vi "preliminaries.vi"(5 "Version":string, 6 "error in":errorcluster, 9 "control cluster":T1) -> (0 "error out":errorcluster, 1 "timing source out":string, 3 "reference cluster out":T2, 4 "error event refnum":refnum<event-registration>)   [LabVIEW 2016]
uses:
  Type Definitions/reference_cluster.ctl
  Type Definitions/vars_settings.ctl
  Type Definitions/stim_type.ctl
  Type Definitions/backlight_type.ctl
  Type Definitions/vars_runtime.ctl
  Type Definitions/data.ctl
  Type Definitions/notifier_elements_GUI.ctl
  Type Definitions/notifier_elements_DAQ.ctl
  Type Definitions/notifier_elements_write.ctl
  Type Definitions/control_references.ctl
  <vilib>/DAQmx/create/timing.llb/DAQmx Create Timing Source (Frequency).vi
types:
  T1 = typedef "control_references.ctl" = cluster{"Base Directory":refnum<vi>, "Config File":refnum<vi>, "Timing Issues":refnum<vi>, "Quit":refnum<vi>, "Animal ID":refnum<vi>[], "Session ID":refnum<vi>[], "Active":refnum<vi>[], "Temperature Charts":refnum<vi>[], "Lick Charts":refnum<vi>[], "Bool Displays":refnum<vi>[], "Stimulus Timing":refnum<vi>[], "Stimulus Stats":refnum<vi>[], "Catch Stats":refnum<vi>[], "Recording Status":refnum<vi>[], "Pairing":refnum<vi>[]}
  T2 = typedef "reference_cluster.ctl" = cluster{"Vars":cluster{"General":refnum<notifier>, "Runtime":refnum<notifier>}, "Data":cluster{"Display":refnum<queue>, "Write":refnum<queue>}, "LoopCtrl":cluster{"Display":refnum<notifier>, "DAQ":refnum<notifier>, "Write":refnum<notifier>[]}, "Controls":T1, "Error Event":refnum<user-event>}
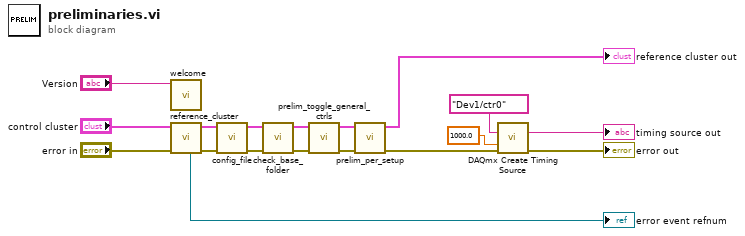
[diagram p0: block diagram]
diagram:
  n1 = call "welcome.vi"("Version"="Version") -> ()  [unwired: 6 in, 1 out]
  n2 = call "reference_cluster.vi"("control cluster"="control cluster", "error in"="error in") -> ("error event refnum"=→"error event refnum":refnum<event-registration>, "reference cluster"=w14:T2, "error out"=w11:errorcluster)  [unwired: 4 in]
  n3 = call "config_file.vi"("error in"=w11, "reference cluster in"=w14) -> ("error out"=w12:errorcluster, "reference cluster out"=w13:T2)  [unwired: 8 in]
  n4 = call "check_base_folder.vi"("error in"=w12, "reference cluster in"=w13) -> ("error out"=w7:errorcluster, "reference cluster out"=w6:T2)  [unwired: 8 in]
  n5 = call "prelim_toggle_general_ctrls.vi"("error in"=w7, "reference cluster"=w6) -> ("error out"=w5:errorcluster, "reference cluster"=w4:T2)  [unwired: 8 in]
  n6 = call "prelim_per_setup.vi"("error in"=w5, "reference cluster"=w4) -> ("error out"=w3:errorcluster, "reference cluster"=→"reference cluster out":T2)  [unwired: 8 in]
  n7 = call-poly <vilib>:"DAQmx Create Timing Source.vi"("counter"=tag "Dev1/ctr0", "frequency"=1000.0, "error in"=w3) -> ("timing source out"=→"timing source out":string, "error out"=→"error out":errorcluster)  [unwired: 11 in]
